vi "Behavior.vi"() -> ()   [LabVIEW 2011]
panel:
  in  "Behavior":string
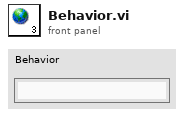
[diagram p1: front panel]
diagram:
